vi "MX1_Powerstage_v1.vi"() -> (3 "Pass/Fail":bool)   [LabVIEW 2022 SP3]
uses:
  <vilib>/DAQmx/read.llb/DAQmx Read (Digital 1D Bool NChan 1Samp 1Line).vi
  <vilib>/DAQmx/miscellaneous.llb/DAQmx Fill In Error Info.vi
panel:
  out "data":bool[](array[boolean])
  out "error out":errorcluster
  in  "error in (no error)":errorcluster
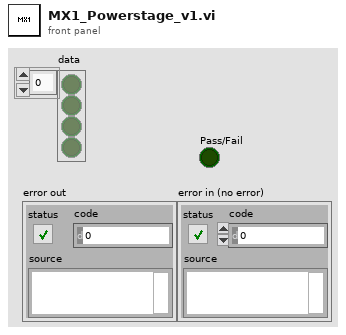
[diagram p1: front panel]
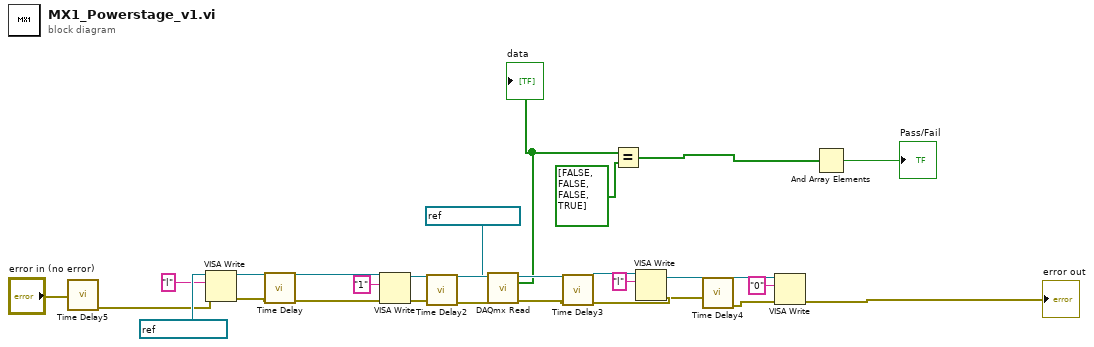
[diagram p0: block diagram]
diagram:
  n1 = call "Time Delay5"("error in (no error)"="error in (no error)") -> ("error out"=w1:errorcluster)  [unwired: 10 in]
  n2 = VISA Write(VISA resource name=refnum<visa-resource-name> "ControlBoard", write buffer="l", error in (no error)=w1) -> (VISA resource name out=w21:refnum<visa-resource-name>, error out=w23:errorcluster)  [unwired: 1 out]
  n3 = call "Time Delay"("error in (no error)"=w23) -> ("error out"=w20:errorcluster)  [unwired: 10 in]
  n4 = VISA Write(VISA resource name=w21, write buffer="1", error in (no error)=w20) -> (VISA resource name out=w17:refnum<visa-resource-name>, error out=w19:errorcluster)  [unwired: 1 out]
  n5 = call "Time Delay2"("error in (no error)"=w19) -> ("error out"=w18:errorcluster)  [unwired: 10 in]
  n6 = call-poly <vilib>:"DAQmx Read.vi"("task/channels in"=refnum<k21> "FTS2_RelayIn", "error in"=w18) -> ("data"=w10:bool[], "error out"=w16:errorcluster)  [unwired: 11 in, 1 out]
  "data" <- w10
  n7 = call "Time Delay3"("error in (no error)"=w16) -> ("error out"=w15:errorcluster)  [unwired: 10 in]
  n8 = Equal?(x=w10, y=bool[] [FALSE, FALSE, FALSE, TRUE]) -> (x = y?=w3:bool[])
  n9 = VISA Write(VISA resource name=w17, write buffer="l", error in (no error)=w15) -> (VISA resource name out=w11:refnum<visa-resource-name>, error out=w13:errorcluster)  [unwired: 1 out]
  n10 = call "Time Delay4"("error in (no error)"=w13) -> ("error out"=w12:errorcluster)  [unwired: 10 in]
  n11 = VISA Write(VISA resource name=w11, write buffer="0", error in (no error)=w12) -> (error out=→"error out":errorcluster)  [unwired: 2 out]
  n12 = And Array Elements(Boolean array=w3) -> (logical AND=→"Pass/Fail":bool)
